vi "Create Time Delayed Send Message.vi"(8 "error in (no error)":errorcluster, 11 "Splash Screen Contract Model in":refnum<class "Splash Screen Contract Model.lvclass">) -> (0 "error out":errorcluster, 3 "Splash Screen Contract Model out":refnum<class "Splash Screen Contract Model.lvclass">)   [LabVIEW 2019, in "Splash Screen Contract Model.lvclass"]
uses:
  <vilib>/gpm_packages/@cs/Car-wash/Source/Splash Screen Contract Model/Splash Screen Contract Model.lvclass
  C:/Program Files/National Instruments/LabVIEW 2019/vi.lib/ActorFramework/Actor/Actor.lvclass
  <vilib>/gpm_packages/@cs/Car-wash/Source/Splash Screen Contract Model Messages/Stop Splash Screen Msg/Stop Splash Screen Msg.lvclass
  C:/Program Files/National Instruments/LabVIEW 2019/vi.lib/ActorFramework/Message/Message.lvclass
  <vilib>/ActorFramework/Actor/Actor.lvclass/Actor.ctl
  <vilib>/ActorFramework/Message Enqueuer/Message Enqueuer.lvclass/Message Enqueuer.ctl
  <vilib>/ActorFramework/Message Enqueuer/Init from Existing Queue.vi
  <vilib>/ActorFramework/Message Enqueuer/Message Enqueuer.lvclass
  <vilib>/ActorFramework/Actor/Actor.lvclass
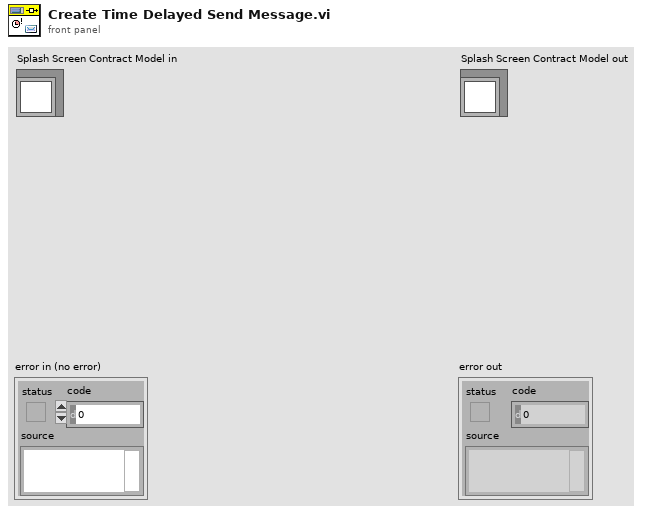
[diagram p1: front panel]
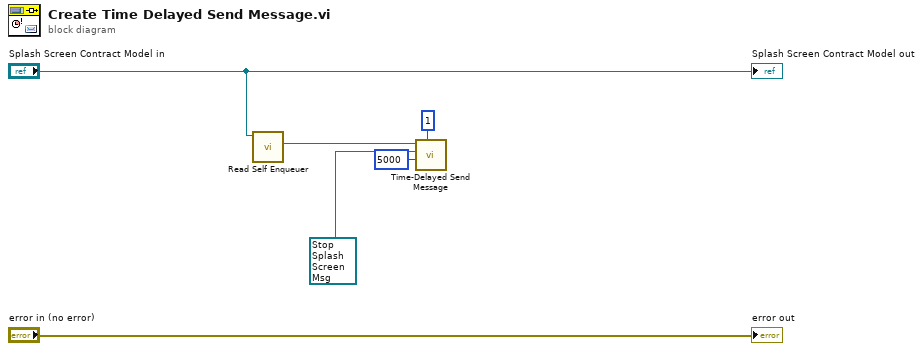
[diagram p0: block diagram]
diagram:
  n1 = call <vilib>:"Read Self Enqueuer.vi"("Actor"="Splash Screen Contract Model in") -> ("Self Enqueuer"=w5:refnum<class "Message Enqueuer.lvclass">)  [unwired: 10 in]
  n2 = call <vilib>:"Time-Delayed Send Message.vi"("# Copies (0 = infinite repeat)"=u32 1, "Milliseconds To Wait"=5000, "Message"=refnum<class "Stop Splash Screen Msg.lvclass"> refnum ("Stop Splash Screen Msg.lvclass"), "Message Enqueuer"=w5) -> ()  [unwired: 6 in, 2 out]
  "error out" <- "error in (no error)"
  "Splash Screen Contract Model out" <- "Splash Screen Contract Model in"
